vi "Cost manage.vi"(8 "error in (no error)":errorcluster, 9 "Cost":u8, 10 "Name":string, 11 "User Interface in":refnum<class "User Interface.lvclass">) -> (0 "error out":errorcluster, 3 "User Interface out":refnum<class "User Interface.lvclass">)   [LabVIEW 2020, in "User Interface.lvlib" / "User Interface.lvclass"]
uses:
  User Interface.lvclass
  C:/Program Files (x86)/National Instruments/LabVIEW 2020/vi.lib/ActorFramework/Actor/Actor.lvclass
  User Interface.lvclass/User Interface.ctl
  <vilib>/ActorFramework/Actor/Actor.lvclass/Actor.ctl
  <vilib>/ActorFramework/Message Enqueuer/Message Enqueuer.lvclass/Message Enqueuer.ctl
  <vilib>/ActorFramework/Message Enqueuer/Init from Existing Queue.vi
  <vilib>/ActorFramework/Message Enqueuer/Enqueue.vi
  User Interface Messages/Validate Purchase Msg/Validate Purchase Msg.lvclass
  C:/Program Files (x86)/National Instruments/LabVIEW 2020/vi.lib/ActorFramework/Message/Message.lvclass
  <vilib>/ActorFramework/Message Priority Queue/Priority Enqueue.vi
  <vilib>/ActorFramework/Message Enqueuer/Message Enqueuer.lvclass
  <vilib>/ActorFramework/Actor/Actor.lvclass
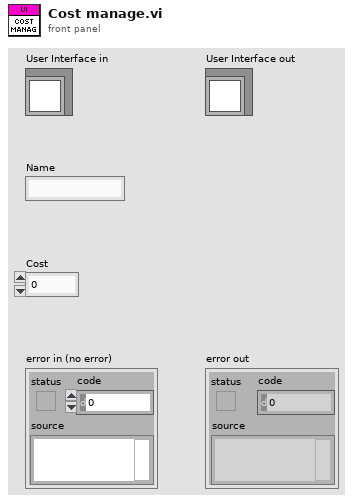
[diagram p1: front panel]
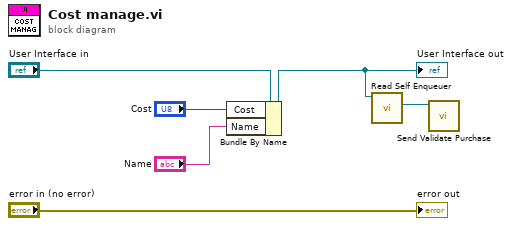
[diagram p0: block diagram]
diagram:
  n1 = Bundle By Name(cluster="User Interface in", "Cost"="Cost", "Name"="Name") -> (w2:refnum<class "User Interface.lvclass">)
  "User Interface out" <- w2
  n2 = call <vilib>:"Read Self Enqueuer.vi"("Actor"=w2) -> ("Self Enqueuer"=w1:refnum<class "Message Enqueuer.lvclass">)  [unwired: 10 in]
  n3 = call "Send Validate Purchase.vi"("Message Enqueuer"=w1) -> ()  [unwired: 9 in, 2 out]
  "error out" <- "error in (no error)"
